vi "Center Text.vi"(8 "error in (no error)":errorcluster, 11 "Dialog in":refnum<class "Dialog.lvclass">) -> (0 "error out":errorcluster, 3 "Dialog out":refnum<class "Dialog.lvclass">)   [LabVIEW 2012, in "Dialog.lvlib" / "Dialog.lvclass"]
uses:
  Dialog.lvclass
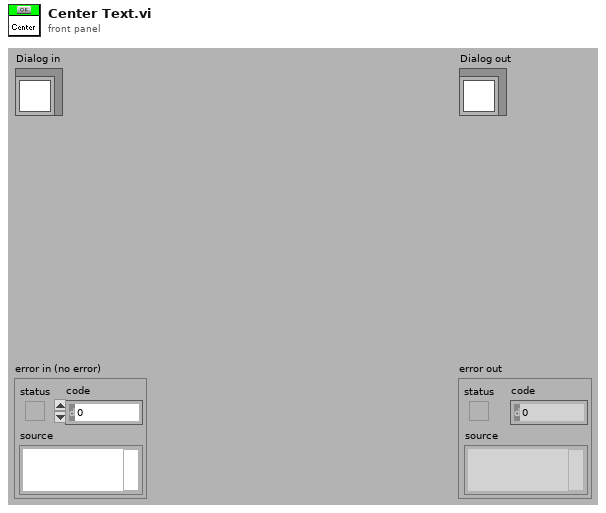
[diagram p1: front panel]
types:
  T1 = cluster{"left":i16, "top":i16, "right":i16, "bottom":i16}
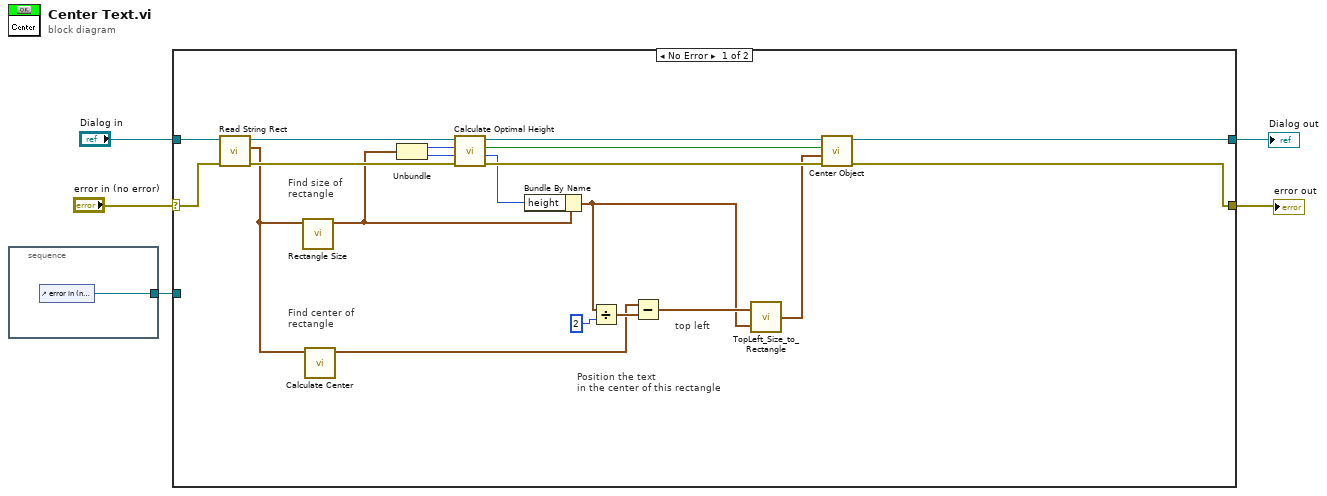
[diagram p0: block diagram]
diagram:
  n1 = stacked-sequence {
    tunnel: [w6] -> w1
    frame #0 {
      n2 = control-ref of="error in (no error)"() -> (w6:refnum<vi>)
    }
  }
  n3 = case shown="No Error" "error in (no error)" {
    selector: "error in (no error)" -> [w16 w28]
    tunnel: [w8 w28] -> w2
    tunnel: [w7 w27] -> w4
    tunnel: "Dialog in" -> [w17 w27]
    tunnel: w1 -> [_ _]
    frame No Error {
      # "top left"
      # "Find size of\nrectangle"
      # "Position the text\nin the center of this rectangle"
      # "Find center of\nrectangle"
      n4 = call-dynamic "Read String Rect.vi"("error in (no error)"=w16, "Dialog.lvclass in"=w17) -> ("error out"=w14:errorcluster, "Object Rect"=w13:T1, "Dialog.lvclass out"=w15:refnum<class "Dialog.lvclass">)  [unwired: 7 out]
      n5 = call "Rectangle Size.vi"("Rectangle"=w13) -> ("Rect Size"=w12:cluster{"width":i32, "height":i32})  [unwired: 10 out]
      n6 = call "Calculate Center.vi"("Rectangle"=w13) -> ("Center"=w25:cluster{"x":i32, "y":i32})  [unwired: 10 out]
      n7 = Unbundle(w12) -> ("width"=w19:i32, "height"=w22:i32)
      n8 = call-dynamic "Calculate Optimal Height.vi"("error in (no error)"=w14, "Max Height (200)"=w22, "Target Width (300)"=w19, "Dialog in"=w15) -> ("error out"=w20:errorcluster, "Set Height"=w18:u32, "VScrollbar Visible?"=w23:bool, "Dialog out"=w21:refnum<class "Dialog.lvclass">)  [unwired: 4 out]
      n9 = Bundle By Name(cluster=w12, "height"=w18) -> (w9:cluster{"width":i32, "height":i32})
      n10 = Divide(x=w9, y=2) -> (x/y=w26:cluster{"width":dbl, "height":dbl})
      n11 = Subtract(x=w25, y=w26) -> (x-y=w11:cluster{dbl, dbl})
      n12 = call "TopLeft_Size_to_Rectangle.vi"("Size"=w9, "Top Left"=w11) -> ("Rectangle"=w10:T1)
      n13 = call-dynamic "Center Object.vi"("error in"=w20, "Rectangle"=w10, "Scrollbar Visible?"=w23, "Dialog in"=w21) -> ("error out"=w8:errorcluster, "Dialog.lvclass out"=w7:refnum<class "Dialog.lvclass">)  [unwired: 6 out]
    }
    frame Error {
    }
  }
  "error out" <- w2
  "Dialog out" <- w4
